vi "SVX Buffer Waterfall Graph (Waterfall Data).vi"(5 "reset on change to dx (F)":bool, 6 "number of spectra (40)":i32=40, 7 "reset? (F)":bool, 8 "error in (no error)":errorcluster, 11 "waterfall graph data":T1={"z0"=0.0, "dz"=1.0, "plots"=[]}) -> (0 "error out":errorcluster, 3 "waterfall graph data out":T1={"z0"=0.0, "dz"=1.0, "plots"=[]})   [LabVIEW 2017, in "SoundVib_SpectralDisplay.lvlib"]
doc: "Buffers signals and returns the buffered signals up to a maximum count. If you use this VI with the Waterfall Graph, the display mimics the behavior of a chart. Wire data to the <B>waterfall graph data</B> input to determine the polymorphic instance to use or manually select the instance."
uses:
  <vilib>/addons/Sound and Vibration/Order Analysis/Data Presentation/SoundVib_SpectralDisplay.lvlib
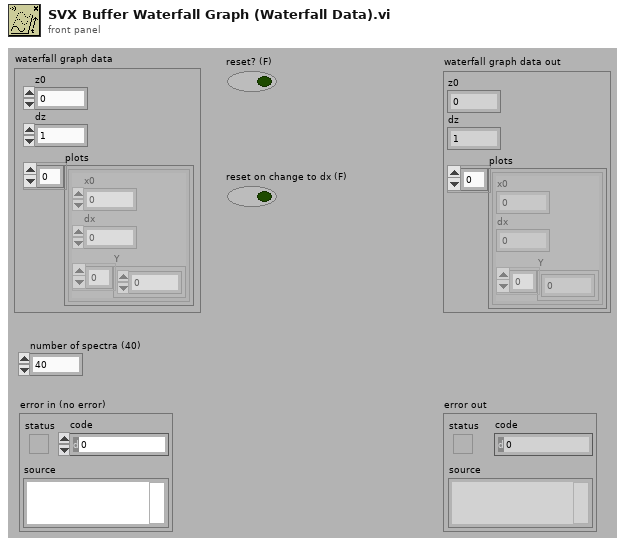
[diagram p1: front panel]
types:
  T1 = cluster{"z0":dbl, "dz":dbl, "plots":cluster{"x0":dbl, "dx":dbl, "Y":dbl[]}[]}
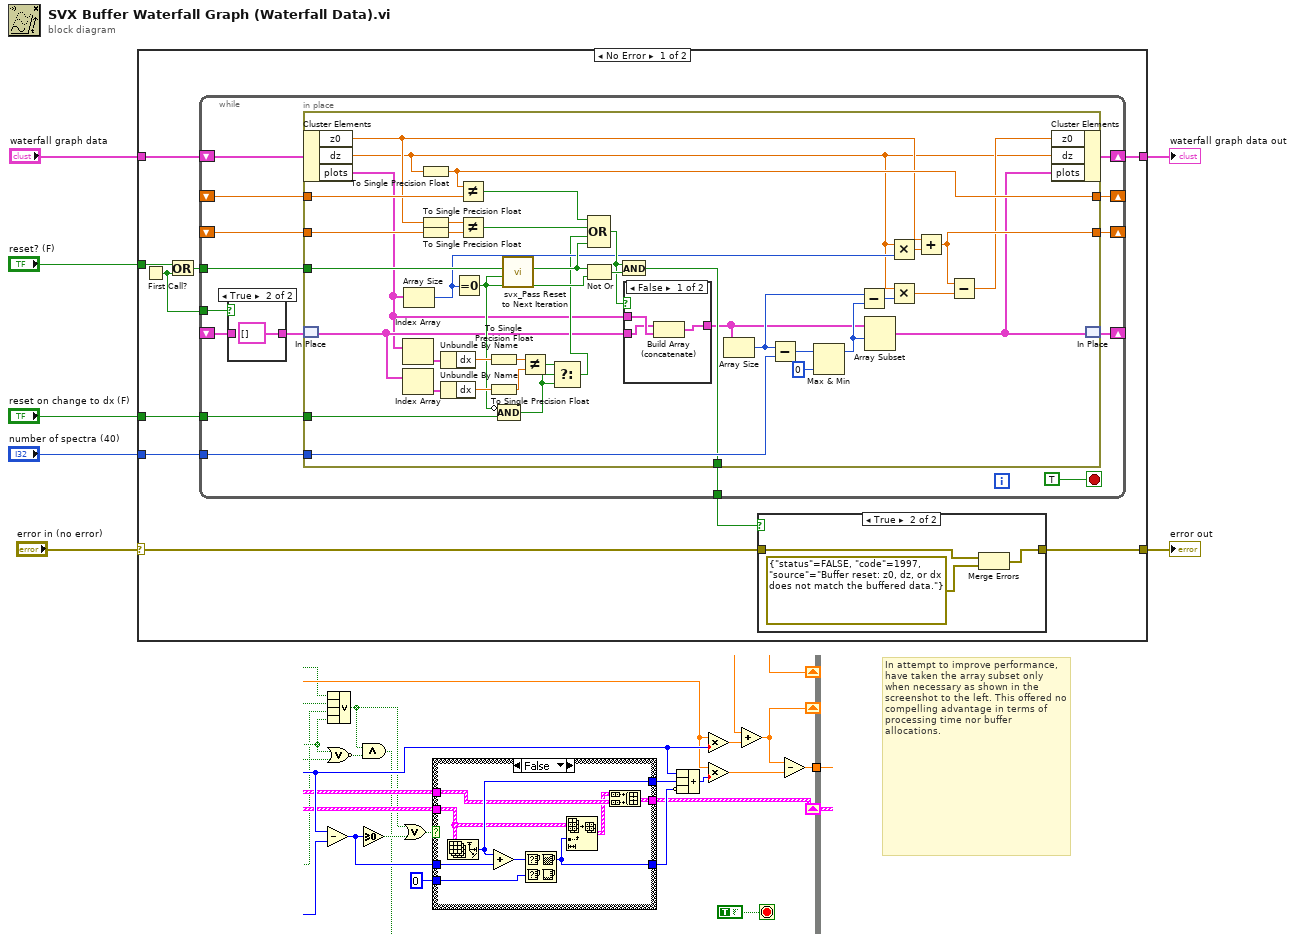
[diagram p0: block diagram]
diagram:
  # "In attempt to improve performance, have taken the array subset only when necessary as shown in the screenshot to the left. This offered no compelling advantage in terms of processing time nor buffer allocations."
  n1 = case shown="No Error" "error in (no error)" {
    selector: "error in (no error)" -> [w16 w84]
    tunnel: [w15 w84] -> w6
    tunnel: "reset? (F)" -> [w13 _]
    tunnel: "number of spectra (40)" -> [w17 _]
    tunnel: "waterfall graph data" -> [w10 w83]
    tunnel: [w9 w83] -> w2
    tunnel: "reset on change to dx (F)" -> [w11 _]
    frame No Error {
      n2 = First Call?() -> (First Call?: T/F=w8:bool)
      n3 = Or(x=w13, y=w8) -> (x .or. y?=w12:bool)
      n4 = while {
        tunnel: w17 -> [w35]
        shift-right: [w25] -> _
        shift-left: _ -> [w23]
        shift-right: [w32] -> _
        shift-left: _ -> [w31]
        shift-right: [w30] -> _
        shift-left: _ -> [w33]
        tunnel: [w34] -> w14
        tunnel: w12 -> [w29]
        tunnel: w11 -> [w28]
        shift-right: [w26] -> w9
        shift-left: w10 -> [w27]
        tunnel: w8 -> [w22]
        stop <- TRUE stop-if-true
        n5 = case shown="True" w22 {
          tunnel: [w37 cluster{"x0":dbl, "dx":dbl, "Y":dbl[]}[] [] ("plots")] -> w24
          tunnel: w23 -> [w37 _]
          frame False {
          }
          frame True {
          }
        }
        n6 = in-place {
          in-place-border: w35 -> [w78]
          in-place-border: [w73] -> w34
          in-place-border: w33 -> [w72]
          in-place-border: [w66] -> w32
          in-place-border: w31 -> [w63]
          in-place-border: [w61] -> w30
          in-place-border: w29 -> [w60]
          in-place-border: w28 -> [w58]
          n7 = in-place-cluster #1(w27) -> ("z0"=w45:dbl, "dz"=w43:dbl, "plots"=w40:cluster{"x0":dbl, "dx":dbl, "Y":dbl[]}[])
          n8 = in-place-match #2(w24) -> (w42:cluster{"x0":dbl, "dx":dbl, "Y":dbl[]}[])
          n9 = Index Array(array=w40) -> (element=w55:cluster{"x0":dbl, "dx":dbl, "Y":dbl[]})  [unwired: 1 in]
          n10 = Index Array(array=w42) -> (element=w54:cluster{"x0":dbl, "dx":dbl, "Y":dbl[]})  [unwired: 1 in]
          n11 = Array Size(array=w40) -> (size(s)=w56:i32)
          n12 = To Single Precision Float(number=w43) -> (single precision float=w61:sgl)
          n13 = To Single Precision Float(number=w45) -> (single precision float=w70:sgl)
          n14 = To Single Precision Float(number=w63) -> (single precision float=w62:sgl)
          n15 = Unbundle By Name(w55) -> ("dx"=w52:dbl)
          n16 = Unbundle By Name(w54) -> ("dx"=w53:dbl)
          n17 = Equal To 0?(x=w56) -> (x = 0?=w47:bool)
          n18 = Not Equal?(x=w61, y=w72) -> (x != y?=w71:bool)
          n19 = Not Equal?(x=w70, y=w62) -> (x != y?=w69:bool)
          n20 = To Single Precision Float(number=w52) -> (single precision float=w51:sgl)
          n21 = To Single Precision Float(number=w53) -> (single precision float=w50:sgl)
          n22 = Compound Arithmetic op=AND(invert w47, w58) -> (w49:bool)
          n23 = call <vilib>:"svx_Pass Reset to Next Iteration.vi"("trigger"=w47, "reset?(F)"=w60) -> ("reset out"=w59:bool)  [unwired: 9 in]
          n24 = Not Equal?(x=w51, y=w50) -> (x != y?=w48:bool)
          n25 = Select(t=w48, s=w49, f=w49) -> (s? t:f=w46:bool)
          n26 = Not Or(1:w47, 2:w59) -> (0:w74:bool)
          n27 = Compound Arithmetic op=OR(w71, w69, w46, w59) -> (w57:bool)
          n28 = And(x=w57, y=w74) -> (x .and. y?=w73:bool)
          n29 = case shown="False" w57 {
            tunnel: [w80 w82] -> w39
            tunnel: w42 -> [w79 _]
            tunnel: w40 -> [w81 w82]
            frame False {
              n30 = Build Array (concatenate)(w79, w81) -> (w80:cluster{"x0":dbl, "dx":dbl, "Y":dbl[]}[])
            }
            frame True {
            }
          }
          n31 = Array Size(array=w39) -> (size(s)=w67:i32)
          n32 = Subtract(x=w67, y=w78) -> (x-y=w77:i32)
          n33 = Max & Min(x=w77, y=0) -> (max(x,y)=w68:i32)  [unwired: 1 out]
          n34 = Subtract(x=w67, y=w68) -> (x-y=w65:i32)
          n35 = Array Subset(array=w39, index=w68) -> (w41:cluster{"x0":dbl, "dx":dbl, "Y":dbl[]}[])  [unwired: 1 in]
          n36 = Multiply(x=w43, y=w56) -> (x*y=w75:dbl)
          n37 = Multiply(x=w43, y=w65) -> (x*y=w64:dbl)
          n38 = Add(x=w45, y=w75) -> (x+y=w66:dbl)
          n39 = Subtract(x=w66, y=w64) -> (x-y=w44:dbl)
          n40 = in-place-cluster #1("z0"=w44, "dz"=w43, "plots"=w41) -> (w26:T1)
          n41 = in-place-match #2(w41) -> (w25:cluster{"x0":dbl, "dx":dbl, "Y":dbl[]}[])
        }
      }
      n42 = case shown="True" w14 {
        tunnel: w16 -> [w18 w20]
        tunnel: [w18 w21] -> w15
        frame False {
        }
        frame True {
          n43 = Merge Errors(w20, errorcluster {"status"=FALSE, "code"=1997, "source"="Buffer reset: z0, dz, or dx does not match the buffered data."} ("error IO")) -> (w21:errorcluster)
        }
      }
    }
    frame Error {
    }
  }
  "waterfall graph data out" <- w2
  "error out" <- w6
